vi "Average Waveforms.vi"(8 "Error In":errorcluster, 9 "Waveforms In":waveform(dbl)[](array[waveform])) -> (0 "Error Out":errorcluster, 1 "Averaged Waveforms":waveform(dbl))   [LabVIEW 2015]
uses:
  <vilib>/Analysis/baseanly.llb/Mean (DBL).vi
  <vilib>/Analysis/NI_AALBase.lvlib
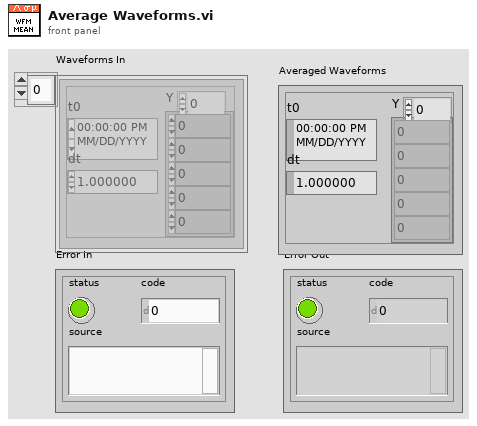
[diagram p1: front panel]
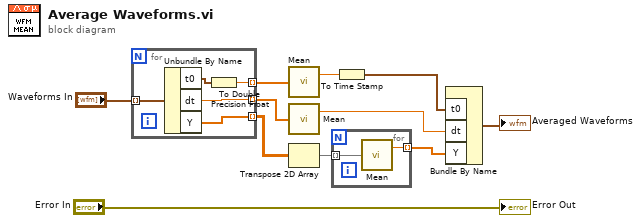
[diagram p0: block diagram]
diagram:
  n1 = for {
    tunnel: "Waveforms In" -> [w16] mode=indexing
    tunnel: [w15] -> w7 mode=indexing
    tunnel: [w14] -> w8 mode=indexing
    tunnel: [w12] -> w5 mode=indexing
    n2 = Unbundle By Name(w16) -> ("t0"=w13:timestamp, "dt"=w15:dbl, "Y"=w14:dbl[])
    n3 = To Double Precision Float(number=w13) -> (double precision float=w12:dbl)
  }
  n4 = call-poly <vilib>:"Mean.vi"("X"=w5) -> ("mean"=w6:dbl)  [unwired: 1 out]
  n5 = call-poly <vilib>:"Mean.vi"("X"=w7) -> ("mean"=w3:dbl)  [unwired: 1 out]
  n6 = Transpose 2D Array(2D array=w8) -> (transposed array=w10:dbl[][])
  n7 = for {
    tunnel: w10 -> [w18] mode=indexing
    tunnel: [w17] -> w11 mode=indexing
    n8 = call-poly <vilib>:"Mean.vi"("X"=w18) -> ("mean"=w17:dbl)  [unwired: 1 out]
  }
  n9 = To Time Stamp(1:w6) -> (0:w4:timestamp)
  n10 = Bundle By Name("t0"=w4, "dt"=w3, "Y"=w11) -> (→"Averaged Waveforms":waveform(dbl))  [unwired: 1 in]
  "Error Out" <- "Error In"
